vi "countrate.vi"() -> ()   [LabVIEW 2015]
uses:
  <vilib>/Platform/TimedLoop/XDataNode/timing_clust.ctl
  <vilib>/Platform/TimedLoop/XDataNode/nitl_modes.ctl
  <vilib>/Platform/TimedLoop/XDataNode/wakeup.ctl
  <vilib>/Utility/file.llb/Write Delimited Spreadsheet (I64).vi
  <vilib>/platform/TimedLoop/XDataNode/XDataNode.xnode
  <vilib>/Platform/TimedLoop/XDataNode/XDNodeRunTimeDep.lvlib
panel:
  in  "Path":path
  out "Waveform Graph":i32[](graph)
  in  "Acusition Time (s)":dbl
  in  "Period (s)":dbl
  out "counts per second":dbl(knob) scale=0.0..100.0
  in  "stop":bool
  # "Demo count rate VI for Physics 434"
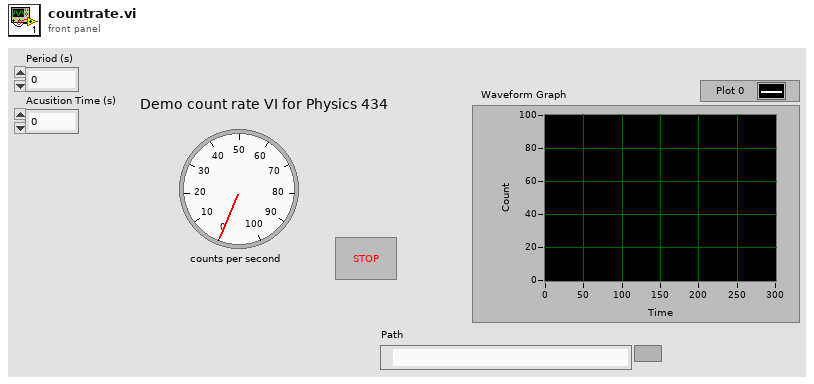
[diagram p1: front panel]
types:
  T1 = typedef "XDNodeRunTimeDep.lvlib/timing_clust.ctl" = cluster{"Expected End [f-1]":u64, "Actual End [f-1]":u64, "Finished Late? [f-1]":bool, "Expected End [i-1]":u64, "Actual End [i-1]":u64, "Finished Late? [i-1]":bool, "Expected Start [i]":u64, "Actual Start [i]":u64, "Expected Start [f]":u64, "Actual Start [f]":u64, "Source Name":string, "Structure Name":string, "Period":i64, "Deadline":i64, "Offset":i64, "Start":i64, "Priority":i32, "Timeout":i32, "Mode":T2, "Wakeup Reason":T3, "Error":errorcluster, "Source Type":string, "Secondary Source Type":string, "Global End Time":u64, "Global Start Time":u64, "Frame Duration":u64, "Iteration Duration":u64, "Assigned CPU":i32, "I/O Scan Engine Mode":u32}
  T2 = typedef "XDNodeRunTimeDep.lvlib/nitl_modes.ctl" = enum32{"No Change", "Process missed periods, maintain original phase", "Discard missed periods, maintain original phase", "Process missed periods, ignore original phase", "Discard missed periods, ignore original phase"}
  T3 = typedef "XDNodeRunTimeDep.lvlib/wakeup.ctl" = enum32{"Normal", "Aborted", "Asynchronous wakeup", "Timing source error", "Timed loop error", "Timeout"}
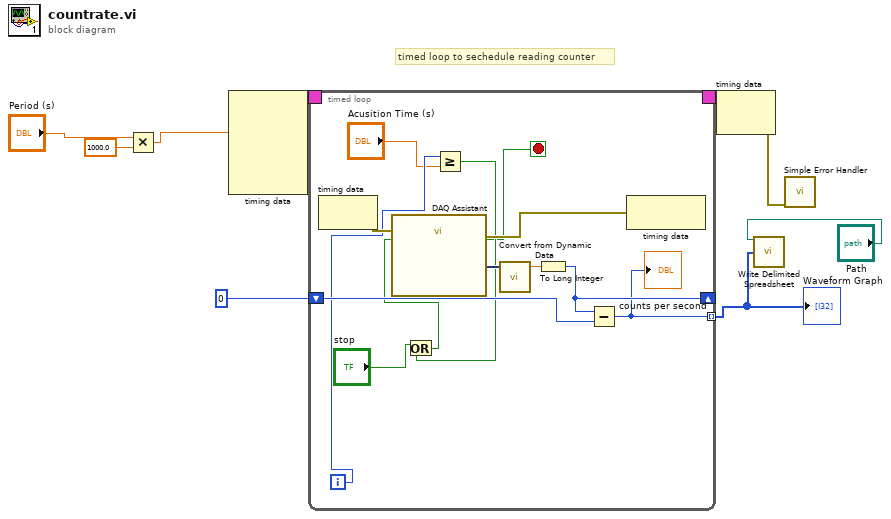
[diagram p0: block diagram]
diagram:
  # "timed loop to sechedule reading counter"
  n1 = Multiply(x="Period (s)", y=1000.0) -> (x*y=w3:dbl)
  n2 = node-c288(w3) -> (w9:T1)  [unwired: 4 in]
  n3 = timed-loop {
    timing: w9 -> [_]
    timing-out: [_] -> w8
    shift-right: [w20] -> _
    shift-left: 0 -> [w21]
    tunnel: [w14] -> w5 mode=indexing
    i -> [w16]
    stop <- w10 stop-if-true
    n4 = node-c288() -> (w17:errorcluster)  [unwired: 1 in]
    n5 = Greater Or Equal?(x=w16, y="Acusition Time (s)") -> (x >= y?=w12:bool)
    n6 = Or(x="stop", y=w12) -> (x .or. y?=w11:bool)
    n7 = call "DAQ Assistant"("error in"=w17, "stop (F)"=w11) -> ("data"=w22:dynamicdata, "stopped"=w10:bool, "error out"=w18:errorcluster)  [unwired: 14 in, 1 out]
    n8 = call "Convert from Dynamic Data"("Dynamic Data Type"=w22) -> ("Scalar"=w19:dbl)  [unwired: 3 in]
    n9 = To Long Integer(number=w19) -> (32bit integer=w20:i32)
    n10 = Subtract(x=w20, y=w21) -> (x-y=w14:i32)
    "counts per second" <- w14
    n11 = node-c288(w18) -> ()  [unwired: 1 out]
  }
  "Waveform Graph" <- w5
  n12 = node-c288(w8) -> (w6:errorcluster)
  n13 = call-poly <vilib>:"Write Delimited Spreadsheet.vi"("file path (dialog if empty)"="Path", "1D data"=w5) -> ()  [unwired: 12 in, 2 out]
  n14 = call <vilib>:"Simple Error Handler.vi"("error in (no error)"=w6) -> ()  [unwired: 4 in, 5 out]
